vi "PS采集测试.vi"() -> ()   [LabVIEW 2020]
uses:
  <vilib>/DAQmx/read.llb/DAQmx Read (Counter 1D DBL 1Chan NSamp).vi
  <vilib>/DAQmx/read.llb/DAQmx Read (Counter DBL 1Chan 1Samp).vi
  <vilib>/DAQmx/create/channels.llb/DAQmx Create Channel (CI-Period).vi
  <vilib>/DAQmx/configure/timing.llb/DAQmx Timing (Implicit).vi
  <vilib>/DAQmx/miscellaneous.llb/DAQmx Fill In Error Info.vi
  <userlib>/_MGI/1D Array/MGI Average/MGI Average (DBL[]).vi
  <vilib>/DAQmx/create/channels.llb/DAQmx Create Channel (CI-Pulse Width).vi
  <resource>/objmgr/daqmx.rc
panel:
  out "周期 8":dbl
  out "周期 7":dbl
  out "周期 6":dbl
  out "周期 5":dbl
  out "周期 4":dbl
  out "周期 3":dbl
  out "占空比 8":dbl
  in  "通道 8":tag="Dev2/ctr7"
  out "占空比 7":dbl
  in  "通道 7":tag="Dev2/ctr6"
  out "占空比 6":dbl
  in  "通道 6":tag="Dev2/ctr5"
  out "占空比 5":dbl
  in  "通道 5":tag="Dev2/ctr4"
  out "占空比 4":dbl
  in  "通道 4":tag="Dev2/ctr3"
  out "占空比 3":dbl
  in  "通道 3":tag="Dev2/ctr2"
  out "周期 2":dbl
  out "占空比 2":dbl
  in  "通道 2":tag="Dev2/ctr1"
  in  "通道":tag="Dev2/ctr0"
  in  "停止":bool
  out "占空比":dbl
  out "周期":dbl
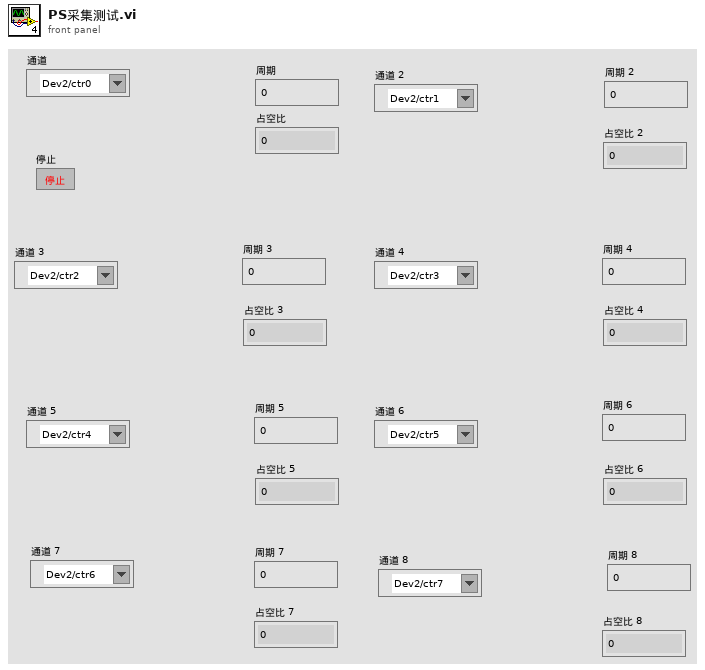
[diagram p1: front panel]
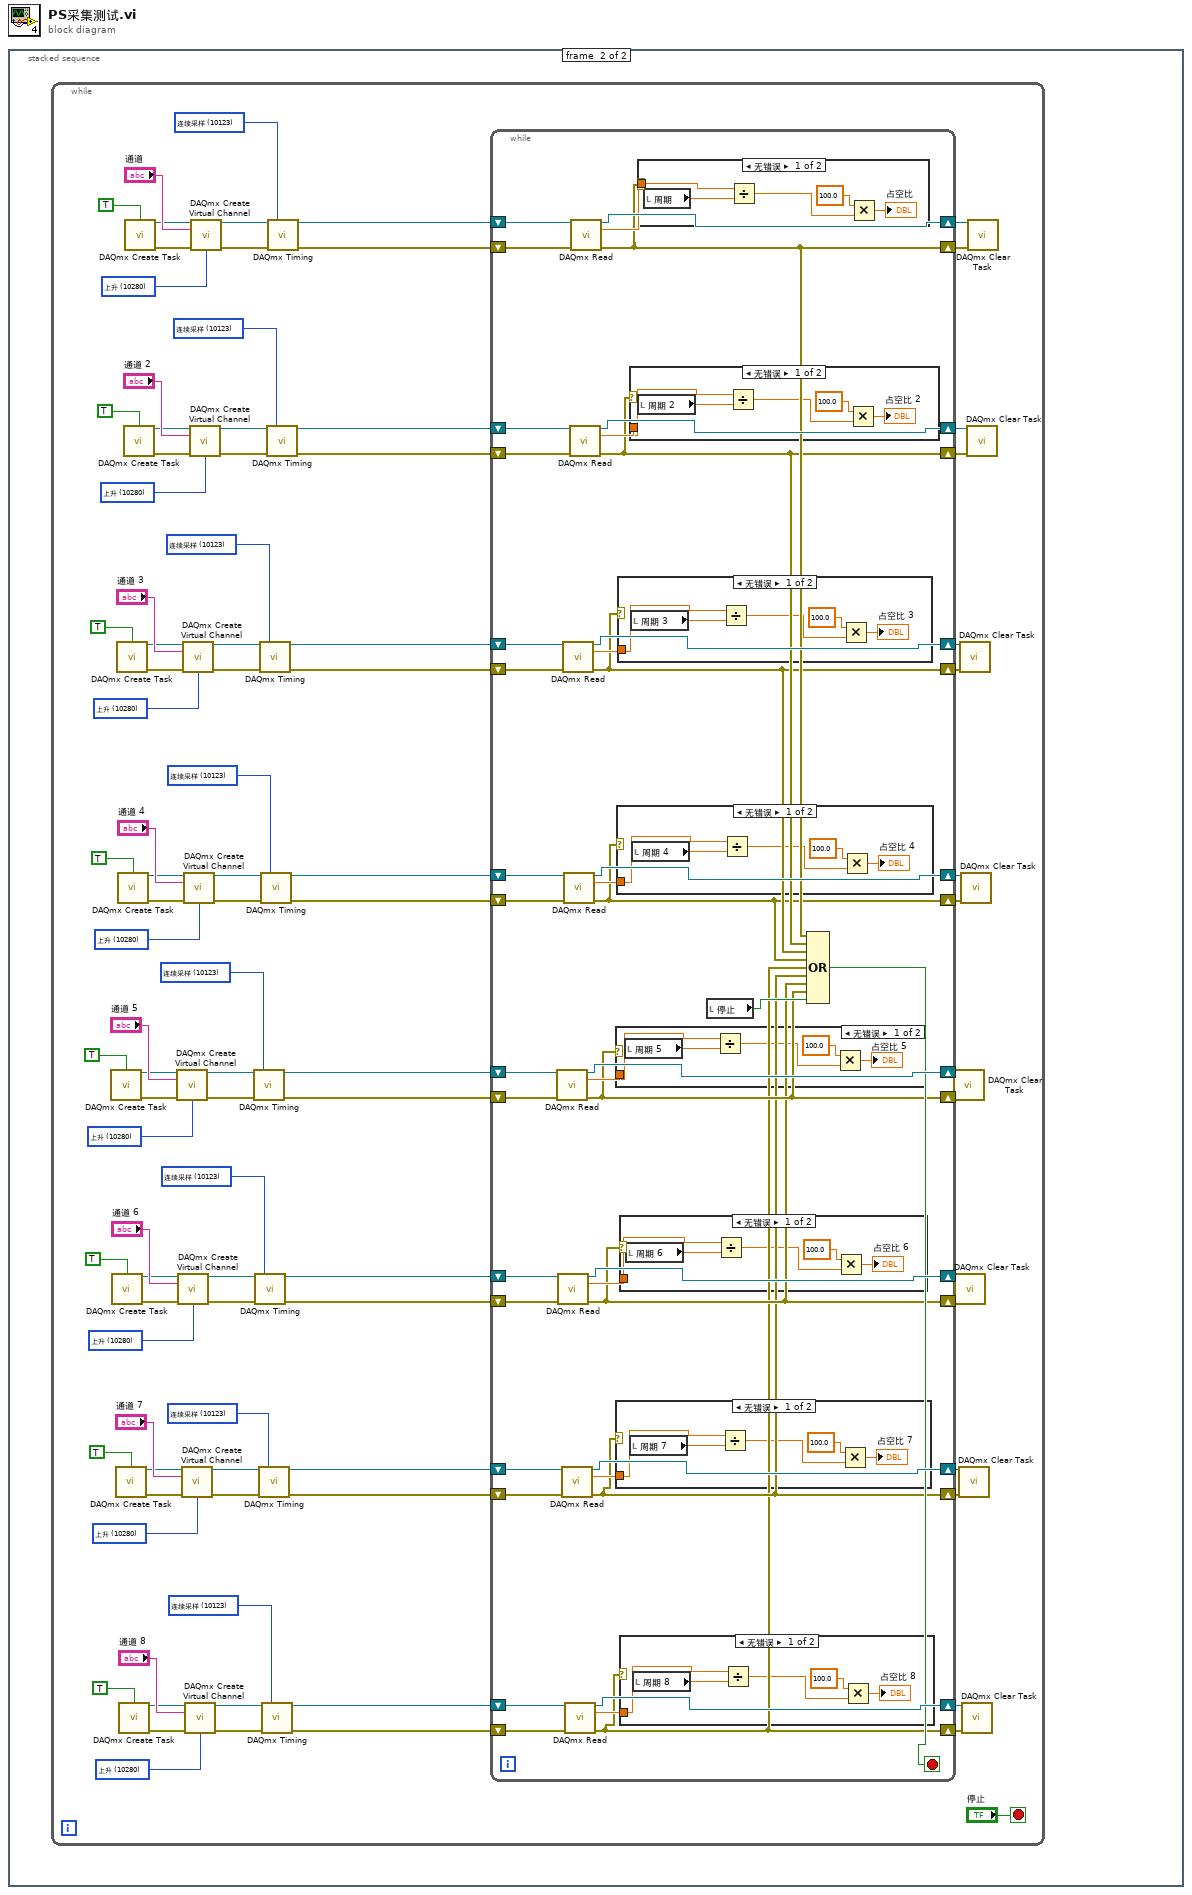
[diagram p0: block diagram]
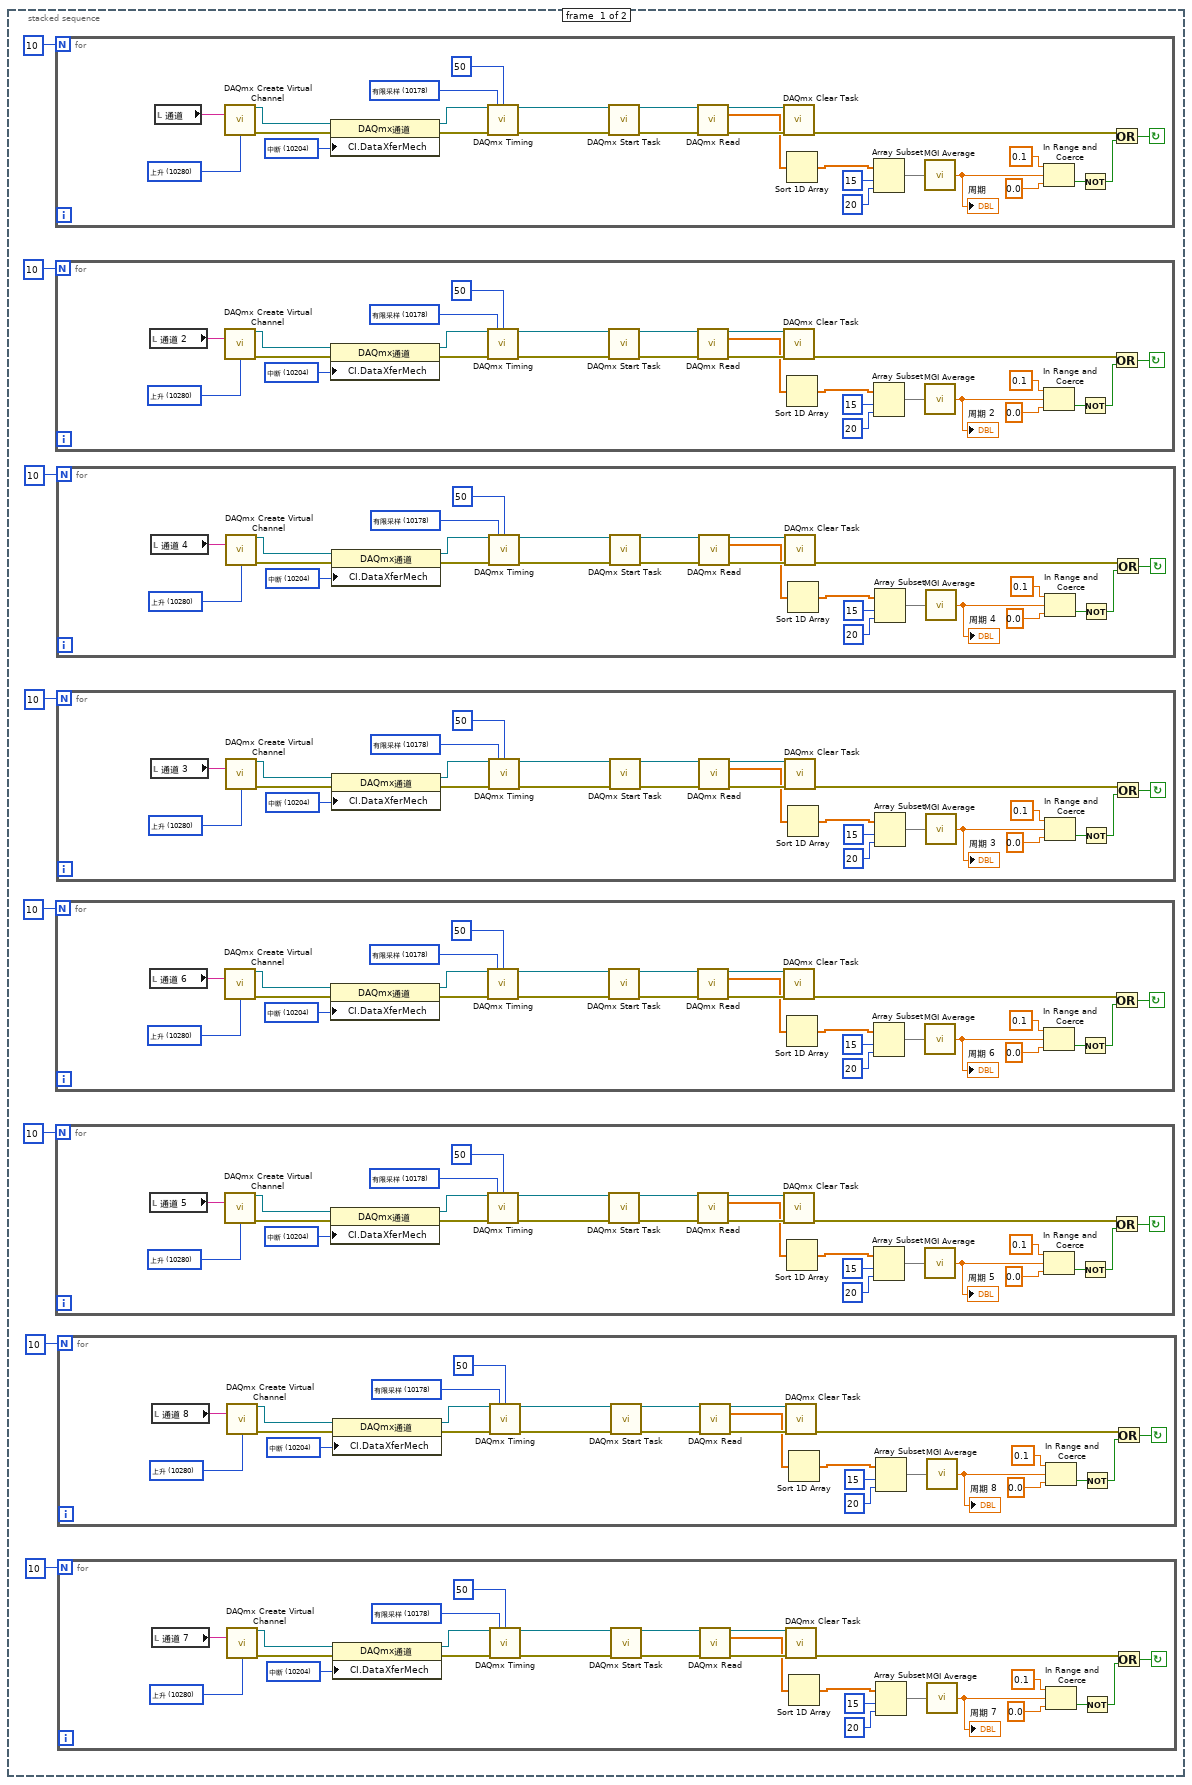
[diagram p2: hidden frame]
diagram:
  n1 = stacked-sequence {
    frame #0 {
      n2 = for {
        N: 10 -> [_]
        stop <- w200 continue-if-true
        w211 = 10204 items=["DMA"=10054, "中断"=10204, "程序控制I/O"=10264, "USB Bulk"=12590] ("CI.DataXferMech")
        w215 = 10178 items=["有限采样"=10178, "连续采样"=10123, "硬件定时单点"=12522] ("sample mode")
        w224 = 10280 items=["上升"=10280, "下降"=10171] ("starting edge")
        n3 = local read "通道"() -> (w198:tag)
        n4 = call-poly <vilib>:"DAQmx Create Virtual Channel.vi"("counter"=w198, "starting edge"=w224) -> ("task out"=w223:refnum<k21>, "error out"=w213:errorcluster)  [unwired: 12 in]
        n5 = property class="DAQmx通道"(reference=w223, error in=w213, "CI.DataXferMech"=w211) -> (reference out=w214:refnum<k21>, error out=w212:errorcluster)
        n6 = call-poly <vilib>:"DAQmx Timing.vi"("task/channels in"=w214, "sample mode"=w215, "samples per channel"=50, "error in"=w212) -> ("task out"=w222:refnum<k21>, "error out"=w221:errorcluster)  [unwired: 10 in]
        n7 = call <vilib>:"DAQmx Start Task.vi"("task/channels in"=w222, "error in"=w221) -> ("task out"=w220:refnum<k21>, "error out"=w219:errorcluster)  [unwired: 12 in]
        n8 = call-poly <vilib>:"DAQmx Read.vi"("task/channels in"=w220, "error in"=w219) -> ("task out"=w217:refnum<k21>, "data"=w207:dbl[], "error out"=w218:errorcluster)  [unwired: 11 in]
        n9 = call <vilib>:"DAQmx Clear Task.vi"("task in"=w217, "error in"=w218) -> ("error out"=w203:errorcluster)  [unwired: 13 in]
        n10 = Sort 1D Array(array=w207) -> (sorted array=w210:dbl[])
        n11 = Array Subset(array=w210, index=15 ("索引"), length=20 ("长度")) -> (w199:dbl[])
        n12 = call-poly <userlib>:"MGI Average.vi"("Double[]"=w199) -> ("Average"=w204:dbl)  [unwired: 1 in]
        "周期" <- w204
        n13 = In Range and Coerce(upper limit=0.1 ("上限"), x=w204, lower limit=0.0 ("上限")) -> (In Range?=w202:bool)  [unwired: 1 out]
        n14 = Not(x=w202) -> (.not. x?=w201:bool)
        n15 = Or(x=w203, y=w201) -> (x .or. y?=w200:bool)
      }
      n16 = for {
        N: 10 -> [_]
        stop <- w173 continue-if-true
        w184 = 10204 items=["DMA"=10054, "中断"=10204, "程序控制I/O"=10264, "USB Bulk"=12590] ("CI.DataXferMech")
        w188 = 10178 items=["有限采样"=10178, "连续采样"=10123, "硬件定时单点"=12522] ("sample mode")
        w197 = 10280 items=["上升"=10280, "下降"=10171] ("starting edge")
        n17 = local read "通道 2"() -> (w171:tag)
        n18 = call-poly <vilib>:"DAQmx Create Virtual Channel.vi"("counter"=w171, "starting edge"=w197) -> ("task out"=w196:refnum<k21>, "error out"=w186:errorcluster)  [unwired: 12 in]
        n19 = property class="DAQmx通道"(reference=w196, error in=w186, "CI.DataXferMech"=w184) -> (reference out=w187:refnum<k21>, error out=w185:errorcluster)
        n20 = call-poly <vilib>:"DAQmx Timing.vi"("task/channels in"=w187, "sample mode"=w188, "samples per channel"=50, "error in"=w185) -> ("task out"=w195:refnum<k21>, "error out"=w194:errorcluster)  [unwired: 10 in]
        n21 = call <vilib>:"DAQmx Start Task.vi"("task/channels in"=w195, "error in"=w194) -> ("task out"=w193:refnum<k21>, "error out"=w192:errorcluster)  [unwired: 12 in]
        n22 = call-poly <vilib>:"DAQmx Read.vi"("task/channels in"=w193, "error in"=w192) -> ("task out"=w190:refnum<k21>, "data"=w180:dbl[], "error out"=w191:errorcluster)  [unwired: 11 in]
        n23 = call <vilib>:"DAQmx Clear Task.vi"("task in"=w190, "error in"=w191) -> ("error out"=w176:errorcluster)  [unwired: 13 in]
        n24 = Sort 1D Array(array=w180) -> (sorted array=w183:dbl[])
        n25 = Array Subset(array=w183, index=15 ("索引"), length=20 ("长度")) -> (w172:dbl[])
        n26 = call-poly <userlib>:"MGI Average.vi"("Double[]"=w172) -> ("Average"=w177:dbl)  [unwired: 1 in]
        "周期 2" <- w177
        n27 = In Range and Coerce(upper limit=0.1 ("上限"), x=w177, lower limit=0.0 ("上限")) -> (In Range?=w175:bool)  [unwired: 1 out]
        n28 = Not(x=w175) -> (.not. x?=w174:bool)
        n29 = Or(x=w176, y=w174) -> (x .or. y?=w173:bool)
      }
      n30 = for {
        N: 10 -> [_]
        stop <- w92 continue-if-true
        w103 = 10204 items=["DMA"=10054, "中断"=10204, "程序控制I/O"=10264, "USB Bulk"=12590] ("CI.DataXferMech")
        w107 = 10178 items=["有限采样"=10178, "连续采样"=10123, "硬件定时单点"=12522] ("sample mode")
        w116 = 10280 items=["上升"=10280, "下降"=10171] ("starting edge")
        n31 = local read "通道 6"() -> (w90:tag)
        n32 = call-poly <vilib>:"DAQmx Create Virtual Channel.vi"("counter"=w90, "starting edge"=w116) -> ("task out"=w115:refnum<k21>, "error out"=w105:errorcluster)  [unwired: 12 in]
        n33 = property class="DAQmx通道"(reference=w115, error in=w105, "CI.DataXferMech"=w103) -> (reference out=w106:refnum<k21>, error out=w104:errorcluster)
        n34 = call-poly <vilib>:"DAQmx Timing.vi"("task/channels in"=w106, "sample mode"=w107, "samples per channel"=50, "error in"=w104) -> ("task out"=w114:refnum<k21>, "error out"=w113:errorcluster)  [unwired: 10 in]
        n35 = call <vilib>:"DAQmx Start Task.vi"("task/channels in"=w114, "error in"=w113) -> ("task out"=w112:refnum<k21>, "error out"=w111:errorcluster)  [unwired: 12 in]
        n36 = call-poly <vilib>:"DAQmx Read.vi"("task/channels in"=w112, "error in"=w111) -> ("task out"=w109:refnum<k21>, "data"=w99:dbl[], "error out"=w110:errorcluster)  [unwired: 11 in]
        n37 = call <vilib>:"DAQmx Clear Task.vi"("task in"=w109, "error in"=w110) -> ("error out"=w95:errorcluster)  [unwired: 13 in]
        n38 = Sort 1D Array(array=w99) -> (sorted array=w102:dbl[])
        n39 = Array Subset(array=w102, index=15 ("索引"), length=20 ("长度")) -> (w91:dbl[])
        n40 = call-poly <userlib>:"MGI Average.vi"("Double[]"=w91) -> ("Average"=w96:dbl)  [unwired: 1 in]
        "周期 6" <- w96
        n41 = In Range and Coerce(upper limit=0.1 ("上限"), x=w96, lower limit=0.0 ("上限")) -> (In Range?=w94:bool)  [unwired: 1 out]
        n42 = Not(x=w94) -> (.not. x?=w93:bool)
        n43 = Or(x=w95, y=w93) -> (x .or. y?=w92:bool)
      }
      n44 = for {
        N: 10 -> [_]
        stop <- w65 continue-if-true
        w76 = 10204 items=["DMA"=10054, "中断"=10204, "程序控制I/O"=10264, "USB Bulk"=12590] ("CI.DataXferMech")
        w80 = 10178 items=["有限采样"=10178, "连续采样"=10123, "硬件定时单点"=12522] ("sample mode")
        w89 = 10280 items=["上升"=10280, "下降"=10171] ("starting edge")
        n45 = local read "通道 5"() -> (w63:tag)
        n46 = call-poly <vilib>:"DAQmx Create Virtual Channel.vi"("counter"=w63, "starting edge"=w89) -> ("task out"=w88:refnum<k21>, "error out"=w78:errorcluster)  [unwired: 12 in]
        n47 = property class="DAQmx通道"(reference=w88, error in=w78, "CI.DataXferMech"=w76) -> (reference out=w79:refnum<k21>, error out=w77:errorcluster)
        n48 = call-poly <vilib>:"DAQmx Timing.vi"("task/channels in"=w79, "sample mode"=w80, "samples per channel"=50, "error in"=w77) -> ("task out"=w87:refnum<k21>, "error out"=w86:errorcluster)  [unwired: 10 in]
        n49 = call <vilib>:"DAQmx Start Task.vi"("task/channels in"=w87, "error in"=w86) -> ("task out"=w85:refnum<k21>, "error out"=w84:errorcluster)  [unwired: 12 in]
        n50 = call-poly <vilib>:"DAQmx Read.vi"("task/channels in"=w85, "error in"=w84) -> ("task out"=w82:refnum<k21>, "data"=w72:dbl[], "error out"=w83:errorcluster)  [unwired: 11 in]
        n51 = call <vilib>:"DAQmx Clear Task.vi"("task in"=w82, "error in"=w83) -> ("error out"=w68:errorcluster)  [unwired: 13 in]
        n52 = Sort 1D Array(array=w72) -> (sorted array=w75:dbl[])
        n53 = Array Subset(array=w75, index=15 ("索引"), length=20 ("长度")) -> (w64:dbl[])
        n54 = call-poly <userlib>:"MGI Average.vi"("Double[]"=w64) -> ("Average"=w69:dbl)  [unwired: 1 in]
        "周期 5" <- w69
        n55 = In Range and Coerce(upper limit=0.1 ("上限"), x=w69, lower limit=0.0 ("上限")) -> (In Range?=w67:bool)  [unwired: 1 out]
        n56 = Not(x=w67) -> (.not. x?=w66:bool)
        n57 = Or(x=w68, y=w66) -> (x .or. y?=w65:bool)
      }
      n58 = for {
        N: 10 -> [_]
        stop <- w146 continue-if-true
        w157 = 10204 items=["DMA"=10054, "中断"=10204, "程序控制I/O"=10264, "USB Bulk"=12590] ("CI.DataXferMech")
        w161 = 10178 items=["有限采样"=10178, "连续采样"=10123, "硬件定时单点"=12522] ("sample mode")
        w170 = 10280 items=["上升"=10280, "下降"=10171] ("starting edge")
        n59 = local read "通道 4"() -> (w144:tag)
        n60 = call-poly <vilib>:"DAQmx Create Virtual Channel.vi"("counter"=w144, "starting edge"=w170) -> ("task out"=w169:refnum<k21>, "error out"=w159:errorcluster)  [unwired: 12 in]
        n61 = property class="DAQmx通道"(reference=w169, error in=w159, "CI.DataXferMech"=w157) -> (reference out=w160:refnum<k21>, error out=w158:errorcluster)
        n62 = call-poly <vilib>:"DAQmx Timing.vi"("task/channels in"=w160, "sample mode"=w161, "samples per channel"=50, "error in"=w158) -> ("task out"=w168:refnum<k21>, "error out"=w167:errorcluster)  [unwired: 10 in]
        n63 = call <vilib>:"DAQmx Start Task.vi"("task/channels in"=w168, "error in"=w167) -> ("task out"=w166:refnum<k21>, "error out"=w165:errorcluster)  [unwired: 12 in]
        n64 = call-poly <vilib>:"DAQmx Read.vi"("task/channels in"=w166, "error in"=w165) -> ("task out"=w163:refnum<k21>, "data"=w153:dbl[], "error out"=w164:errorcluster)  [unwired: 11 in]
        n65 = call <vilib>:"DAQmx Clear Task.vi"("task in"=w163, "error in"=w164) -> ("error out"=w149:errorcluster)  [unwired: 13 in]
        n66 = Sort 1D Array(array=w153) -> (sorted array=w156:dbl[])
        n67 = Array Subset(array=w156, index=15 ("索引"), length=20 ("长度")) -> (w145:dbl[])
        n68 = call-poly <userlib>:"MGI Average.vi"("Double[]"=w145) -> ("Average"=w150:dbl)  [unwired: 1 in]
        "周期 4" <- w150
        n69 = In Range and Coerce(upper limit=0.1 ("上限"), x=w150, lower limit=0.0 ("上限")) -> (In Range?=w148:bool)  [unwired: 1 out]
        n70 = Not(x=w148) -> (.not. x?=w147:bool)
        n71 = Or(x=w149, y=w147) -> (x .or. y?=w146:bool)
      }
      n72 = for {
        N: 10 -> [_]
        stop <- w119 continue-if-true
        w130 = 10204 items=["DMA"=10054, "中断"=10204, "程序控制I/O"=10264, "USB Bulk"=12590] ("CI.DataXferMech")
        w134 = 10178 items=["有限采样"=10178, "连续采样"=10123, "硬件定时单点"=12522] ("sample mode")
        w143 = 10280 items=["上升"=10280, "下降"=10171] ("starting edge")
        n73 = local read "通道 3"() -> (w117:tag)
        n74 = call-poly <vilib>:"DAQmx Create Virtual Channel.vi"("counter"=w117, "starting edge"=w143) -> ("task out"=w142:refnum<k21>, "error out"=w132:errorcluster)  [unwired: 12 in]
        n75 = property class="DAQmx通道"(reference=w142, error in=w132, "CI.DataXferMech"=w130) -> (reference out=w133:refnum<k21>, error out=w131:errorcluster)
        n76 = call-poly <vilib>:"DAQmx Timing.vi"("task/channels in"=w133, "sample mode"=w134, "samples per channel"=50, "error in"=w131) -> ("task out"=w141:refnum<k21>, "error out"=w140:errorcluster)  [unwired: 10 in]
        n77 = call <vilib>:"DAQmx Start Task.vi"("task/channels in"=w141, "error in"=w140) -> ("task out"=w139:refnum<k21>, "error out"=w138:errorcluster)  [unwired: 12 in]
        n78 = call-poly <vilib>:"DAQmx Read.vi"("task/channels in"=w139, "error in"=w138) -> ("task out"=w136:refnum<k21>, "data"=w126:dbl[], "error out"=w137:errorcluster)  [unwired: 11 in]
        n79 = call <vilib>:"DAQmx Clear Task.vi"("task in"=w136, "error in"=w137) -> ("error out"=w122:errorcluster)  [unwired: 13 in]
        n80 = Sort 1D Array(array=w126) -> (sorted array=w129:dbl[])
        n81 = Array Subset(array=w129, index=15 ("索引"), length=20 ("长度")) -> (w118:dbl[])
        n82 = call-poly <userlib>:"MGI Average.vi"("Double[]"=w118) -> ("Average"=w123:dbl)  [unwired: 1 in]
        "周期 3" <- w123
        n83 = In Range and Coerce(upper limit=0.1 ("上限"), x=w123, lower limit=0.0 ("上限")) -> (In Range?=w121:bool)  [unwired: 1 out]
        n84 = Not(x=w121) -> (.not. x?=w120:bool)
        n85 = Or(x=w122, y=w120) -> (x .or. y?=w119:bool)
      }
      n86 = for {
        N: 10 -> [_]
        stop <- w38 continue-if-true
        w49 = 10204 items=["DMA"=10054, "中断"=10204, "程序控制I/O"=10264, "USB Bulk"=12590] ("CI.DataXferMech")
        w53 = 10178 items=["有限采样"=10178, "连续采样"=10123, "硬件定时单点"=12522] ("sample mode")
        w62 = 10280 items=["上升"=10280, "下降"=10171] ("starting edge")
        n87 = local read "通道 8"() -> (w36:tag)
        n88 = call-poly <vilib>:"DAQmx Create Virtual Channel.vi"("counter"=w36, "starting edge"=w62) -> ("task out"=w61:refnum<k21>, "error out"=w51:errorcluster)  [unwired: 12 in]
        n89 = property class="DAQmx通道"(reference=w61, error in=w51, "CI.DataXferMech"=w49) -> (reference out=w52:refnum<k21>, error out=w50:errorcluster)
        n90 = call-poly <vilib>:"DAQmx Timing.vi"("task/channels in"=w52, "sample mode"=w53, "samples per channel"=50, "error in"=w50) -> ("task out"=w60:refnum<k21>, "error out"=w59:errorcluster)  [unwired: 10 in]
        n91 = call <vilib>:"DAQmx Start Task.vi"("task/channels in"=w60, "error in"=w59) -> ("task out"=w58:refnum<k21>, "error out"=w57:errorcluster)  [unwired: 12 in]
        n92 = call-poly <vilib>:"DAQmx Read.vi"("task/channels in"=w58, "error in"=w57) -> ("task out"=w55:refnum<k21>, "data"=w45:dbl[], "error out"=w56:errorcluster)  [unwired: 11 in]
        n93 = call <vilib>:"DAQmx Clear Task.vi"("task in"=w55, "error in"=w56) -> ("error out"=w41:errorcluster)  [unwired: 13 in]
        n94 = Sort 1D Array(array=w45) -> (sorted array=w48:dbl[])
        n95 = Array Subset(array=w48, index=15 ("索引"), length=20 ("长度")) -> (w37:dbl[])
        n96 = call-poly <userlib>:"MGI Average.vi"("Double[]"=w37) -> ("Average"=w42:dbl)  [unwired: 1 in]
        "周期 8" <- w42
        n97 = In Range and Coerce(upper limit=0.1 ("上限"), x=w42, lower limit=0.0 ("上限")) -> (In Range?=w40:bool)  [unwired: 1 out]
        n98 = Not(x=w40) -> (.not. x?=w39:bool)
        n99 = Or(x=w41, y=w39) -> (x .or. y?=w38:bool)
      }
      n100 = for {
        N: 10 -> [_]
        stop <- w11 continue-if-true
        w22 = 10204 items=["DMA"=10054, "中断"=10204, "程序控制I/O"=10264, "USB Bulk"=12590] ("CI.DataXferMech")
        w26 = 10178 items=["有限采样"=10178, "连续采样"=10123, "硬件定时单点"=12522] ("sample mode")
        w35 = 10280 items=["上升"=10280, "下降"=10171] ("starting edge")
        n101 = local read "通道 7"() -> (w9:tag)
        n102 = call-poly <vilib>:"DAQmx Create Virtual Channel.vi"("counter"=w9, "starting edge"=w35) -> ("task out"=w34:refnum<k21>, "error out"=w24:errorcluster)  [unwired: 12 in]
        n103 = property class="DAQmx通道"(reference=w34, error in=w24, "CI.DataXferMech"=w22) -> (reference out=w25:refnum<k21>, error out=w23:errorcluster)
        n104 = call-poly <vilib>:"DAQmx Timing.vi"("task/channels in"=w25, "sample mode"=w26, "samples per channel"=50, "error in"=w23) -> ("task out"=w33:refnum<k21>, "error out"=w32:errorcluster)  [unwired: 10 in]
        n105 = call <vilib>:"DAQmx Start Task.vi"("task/channels in"=w33, "error in"=w32) -> ("task out"=w31:refnum<k21>, "error out"=w30:errorcluster)  [unwired: 12 in]
        n106 = call-poly <vilib>:"DAQmx Read.vi"("task/channels in"=w31, "error in"=w30) -> ("task out"=w28:refnum<k21>, "data"=w18:dbl[], "error out"=w29:errorcluster)  [unwired: 11 in]
        n107 = call <vilib>:"DAQmx Clear Task.vi"("task in"=w28, "error in"=w29) -> ("error out"=w14:errorcluster)  [unwired: 13 in]
        n108 = Sort 1D Array(array=w18) -> (sorted array=w21:dbl[])
        n109 = Array Subset(array=w21, index=15 ("索引"), length=20 ("长度")) -> (w10:dbl[])
        n110 = call-poly <userlib>:"MGI Average.vi"("Double[]"=w10) -> ("Average"=w15:dbl)  [unwired: 1 in]
        "周期 7" <- w15
        n111 = In Range and Coerce(upper limit=0.1 ("上限"), x=w15, lower limit=0.0 ("上限")) -> (In Range?=w13:bool)  [unwired: 1 out]
        n112 = Not(x=w13) -> (.not. x?=w12:bool)
        n113 = Or(x=w14, y=w12) -> (x .or. y?=w11:bool)
      }
    }
    frame #1 {
      n114 = while {
        stop <- "停止" stop-if-true
        w231 = 10123 items=["有限采样"=10178, "连续采样"=10123, "硬件定时单点"=12522] ("sample mode")
        w230 = 10280 items=["上升"=10280, "下降"=10171] ("starting edge")
        w243 = 10123 items=["有限采样"=10178, "连续采样"=10123, "硬件定时单点"=12522] ("sample mode")
        w242 = 10280 items=["上升"=10280, "下降"=10171] ("starting edge")
        w255 = 10123 items=["有限采样"=10178, "连续采样"=10123, "硬件定时单点"=12522] ("sample mode")
        w254 = 10280 items=["上升"=10280, "下降"=10171] ("starting edge")
        w267 = 10123 items=["有限采样"=10178, "连续采样"=10123, "硬件定时单点"=12522] ("sample mode")
        w266 = 10280 items=["上升"=10280, "下降"=10171] ("starting edge")
        w279 = 10123 items=["有限采样"=10178, "连续采样"=10123, "硬件定时单点"=12522] ("sample mode")
        w278 = 10280 items=["上升"=10280, "下降"=10171] ("starting edge")
        w291 = 10123 items=["有限采样"=10178, "连续采样"=10123, "硬件定时单点"=12522] ("sample mode")
        w290 = 10280 items=["上升"=10280, "下降"=10171] ("starting edge")
        w303 = 10123 items=["有限采样"=10178, "连续采样"=10123, "硬件定时单点"=12522] ("sample mode")
        w302 = 10280 items=["上升"=10280, "下降"=10171] ("starting edge")
        w315 = 10123 items=["有限采样"=10178, "连续采样"=10123, "硬件定时单点"=12522] ("sample mode")
        w314 = 10280 items=["上升"=10280, "下降"=10171] ("starting edge")
        n115 = call <vilib>:"DAQmx Create Task.vi"("auto cleanup"=TRUE) -> ("task out"=w252:refnum<k21>, "error out"=w250:errorcluster)  [unwired: 13 in]
        n116 = call <vilib>:"DAQmx Create Task.vi"("auto cleanup"=TRUE) -> ("task out"=w264:refnum<k21>, "error out"=w262:errorcluster)  [unwired: 13 in]
        n117 = call <vilib>:"DAQmx Create Task.vi"("auto cleanup"=TRUE) -> ("task out"=w228:refnum<k21>, "error out"=w226:errorcluster)  [unwired: 13 in]
        n118 = call <vilib>:"DAQmx Create Task.vi"("auto cleanup"=TRUE) -> ("task out"=w288:refnum<k21>, "error out"=w286:errorcluster)  [unwired: 13 in]
        n119 = call <vilib>:"DAQmx Create Task.vi"("auto cleanup"=TRUE) -> ("task out"=w276:refnum<k21>, "error out"=w274:errorcluster)  [unwired: 13 in]
        n120 = call <vilib>:"DAQmx Create Task.vi"("auto cleanup"=TRUE) -> ("task out"=w240:refnum<k21>, "error out"=w238:errorcluster)  [unwired: 13 in]
        n121 = call <vilib>:"DAQmx Create Task.vi"("auto cleanup"=TRUE) -> ("task out"=w300:refnum<k21>, "error out"=w298:errorcluster)  [unwired: 13 in]
        n122 = call <vilib>:"DAQmx Create Task.vi"("auto cleanup"=TRUE) -> ("task out"=w312:refnum<k21>, "error out"=w310:errorcluster)  [unwired: 13 in]
        n123 = call-poly <vilib>:"DAQmx Create Virtual Channel.vi"("task in"=w252, "counter"="通道 5", "error in"=w250, "starting edge"=w254) -> ("task out"=w256:refnum<k21>, "error out"=w261:errorcluster)  [unwired: 10 in]
        n124 = call-poly <vilib>:"DAQmx Create Virtual Channel.vi"("task in"=w264, "counter"="通道 6", "error in"=w262, "starting edge"=w266) -> ("task out"=w268:refnum<k21>, "error out"=w273:errorcluster)  [unwired: 10 in]
        n125 = call-poly <vilib>:"DAQmx Create Virtual Channel.vi"("task in"=w228, "counter"="通道 7", "error in"=w226, "starting edge"=w230) -> ("task out"=w232:refnum<k21>, "error out"=w237:errorcluster)  [unwired: 10 in]
        n126 = call-poly <vilib>:"DAQmx Create Virtual Channel.vi"("task in"=w288, "counter"="通道 3", "error in"=w286, "starting edge"=w290) -> ("task out"=w292:refnum<k21>, "error out"=w297:errorcluster)  [unwired: 10 in]
        n127 = call-poly <vilib>:"DAQmx Create Virtual Channel.vi"("task in"=w276, "counter"="通道 4", "error in"=w274, "starting edge"=w278) -> ("task out"=w280:refnum<k21>, "error out"=w285:errorcluster)  [unwired: 10 in]
        n128 = call-poly <vilib>:"DAQmx Create Virtual Channel.vi"("task in"=w240, "counter"="通道 8", "error in"=w238, "starting edge"=w242) -> ("task out"=w244:refnum<k21>, "error out"=w249:errorcluster)  [unwired: 10 in]
        n129 = call-poly <vilib>:"DAQmx Create Virtual Channel.vi"("task in"=w300, "counter"="通道 2", "error in"=w298, "starting edge"=w302) -> ("task out"=w304:refnum<k21>, "error out"=w309:errorcluster)  [unwired: 10 in]
        n130 = call-poly <vilib>:"DAQmx Create Virtual Channel.vi"("task in"=w312, "counter"="通道", "error in"=w310, "starting edge"=w314) -> ("task out"=w316:refnum<k21>, "error out"=w321:errorcluster)  [unwired: 10 in]
        n131 = call-poly <vilib>:"DAQmx Timing.vi"("task/channels in"=w256, "sample mode"=w255, "error in"=w261) -> ("task out"=w257:refnum<k21>, "error out"=w258:errorcluster)  [unwired: 11 in]
        n132 = call-poly <vilib>:"DAQmx Timing.vi"("task/channels in"=w268, "sample mode"=w267, "error in"=w273) -> ("task out"=w269:refnum<k21>, "error out"=w270:errorcluster)  [unwired: 11 in]
        n133 = call-poly <vilib>:"DAQmx Timing.vi"("task/channels in"=w232, "sample mode"=w231, "error in"=w237) -> ("task out"=w233:refnum<k21>, "error out"=w234:errorcluster)  [unwired: 11 in]
        n134 = call-poly <vilib>:"DAQmx Timing.vi"("task/channels in"=w292, "sample mode"=w291, "error in"=w297) -> ("task out"=w293:refnum<k21>, "error out"=w294:errorcluster)  [unwired: 11 in]
        n135 = call-poly <vilib>:"DAQmx Timing.vi"("task/channels in"=w280, "sample mode"=w279, "error in"=w285) -> ("task out"=w281:refnum<k21>, "error out"=w282:errorcluster)  [unwired: 11 in]
        n136 = call-poly <vilib>:"DAQmx Timing.vi"("task/channels in"=w244, "sample mode"=w243, "error in"=w249) -> ("task out"=w245:refnum<k21>, "error out"=w246:errorcluster)  [unwired: 11 in]
        n137 = call-poly <vilib>:"DAQmx Timing.vi"("task/channels in"=w304, "sample mode"=w303, "error in"=w309) -> ("task out"=w305:refnum<k21>, "error out"=w306:errorcluster)  [unwired: 11 in]
        n138 = call-poly <vilib>:"DAQmx Timing.vi"("task/channels in"=w316, "sample mode"=w315, "error in"=w321) -> ("task out"=w317:refnum<k21>, "error out"=w318:errorcluster)  [unwired: 11 in]
        n139 = while {
          shift-right: [w329] -> w319
          shift-left: w318 -> [w362]
          shift-right: [w363] -> w320
          shift-left: w317 -> [w361]
          shift-right: [w328] -> w307
          shift-left: w306 -> [w359]
          shift-right: [w360] -> w308
          shift-left: w305 -> [w358]
          shift-right: [w327] -> w295
          shift-left: w294 -> [w356]
          shift-right: [w357] -> w296
          shift-left: w293 -> [w355]
          shift-right: [w326] -> w283
          shift-left: w282 -> [w353]
          shift-right: [w354] -> w284
          shift-left: w281 -> [w352]
          shift-right: [w324] -> w271
          shift-left: w270 -> [w350]
          shift-right: [w351] -> w272
          shift-left: w269 -> [w349]
          shift-right: [w325] -> w259
          shift-left: w258 -> [w347]
          shift-right: [w348] -> w260
          shift-left: w257 -> [w346]
          shift-right: [w322] -> w247
          shift-left: w246 -> [w344]
          shift-right: [w345] -> w248
          shift-left: w245 -> [w343]
          shift-right: [w323] -> w235
          shift-left: w234 -> [w341]
          shift-right: [w342] -> w236
          shift-left: w233 -> [w340]
          stop <- w330 stop-if-true
          n140 = call-poly <vilib>:"DAQmx Read.vi"("task/channels in"=w346, "error in"=w347) -> ("task out"=w348:refnum<k21>, "data"=w334:dbl, "error out"=w325:errorcluster)  [unwired: 11 in]
          n141 = call-poly <vilib>:"DAQmx Read.vi"("task/channels in"=w349, "error in"=w350) -> ("task out"=w351:refnum<k21>, "data"=w335:dbl, "error out"=w324:errorcluster)  [unwired: 11 in]
          n142 = call-poly <vilib>:"DAQmx Read.vi"("task/channels in"=w340, "error in"=w341) -> ("task out"=w342:refnum<k21>, "data"=w332:dbl, "error out"=w323:errorcluster)  [unwired: 11 in]
          n143 = call-poly <vilib>:"DAQmx Read.vi"("task/channels in"=w355, "error in"=w356) -> ("task out"=w357:refnum<k21>, "data"=w337:dbl, "error out"=w327:errorcluster)  [unwired: 11 in]
          n144 = call-poly <vilib>:"DAQmx Read.vi"("task/channels in"=w352, "error in"=w353) -> ("task out"=w354:refnum<k21>, "data"=w336:dbl, "error out"=w326:errorcluster)  [unwired: 11 in]
          n145 = call-poly <vilib>:"DAQmx Read.vi"("task/channels in"=w343, "error in"=w344) -> ("task out"=w345:refnum<k21>, "data"=w333:dbl, "error out"=w322:errorcluster)  [unwired: 11 in]
          n146 = call-poly <vilib>:"DAQmx Read.vi"("task/channels in"=w358, "error in"=w359) -> ("task out"=w360:refnum<k21>, "data"=w338:dbl, "error out"=w328:errorcluster)  [unwired: 11 in]
          n147 = call-poly <vilib>:"DAQmx Read.vi"("task/channels in"=w361, "error in"=w362) -> ("task out"=w363:refnum<k21>, "data"=w339:dbl, "error out"=w329:errorcluster)  [unwired: 11 in]
          n148 = case shown="无错误" w325 {
            tunnel: w334 -> [w383 _]
            frame No Error {
              n149 = local read "周期 5"() -> (w382:dbl)
              n150 = Divide(x=w383, y=w382) -> (x/y=w381:dbl)
              n151 = Multiply(x=100.0, y=w381) -> (x*y=→"占空比 5":dbl)
            }
            frame Error {
            }
          }
          n152 = case shown="无错误" w323 {
            tunnel: w332 -> [w373 _]
            frame No Error {
              n153 = local read "周期 7"() -> (w372:dbl)
              n154 = Divide(x=w373, y=w372) -> (x/y=w371:dbl)
              n155 = Multiply(x=100.0, y=w371) -> (x*y=→"占空比 7":dbl)
            }
            frame Error {
            }
          }
          n156 = case shown="无错误" w326 {
            tunnel: w336 -> [w388 _]
            frame No Error {
              n157 = local read "周期 4"() -> (w387:dbl)
              n158 = Divide(x=w388, y=w387) -> (x/y=w386:dbl)
              n159 = Multiply(x=100.0, y=w386) -> (x*y=→"占空比 4":dbl)
            }
            frame Error {
            }
          }
          n160 = case shown="无错误" w327 {
            tunnel: w337 -> [w393 _]
            frame No Error {
              n161 = local read "周期 3"() -> (w392:dbl)
              n162 = Divide(x=w393, y=w392) -> (x/y=w391:dbl)
              n163 = Multiply(x=100.0, y=w391) -> (x*y=→"占空比 3":dbl)
            }
            frame Error {
            }
          }
          n164 = case shown="无错误" w324 {
            tunnel: w335 -> [w378 _]
            frame No Error {
              n165 = local read "周期 6"() -> (w377:dbl)
              n166 = Divide(x=w378, y=w377) -> (x/y=w376:dbl)
              n167 = Multiply(x=100.0, y=w376) -> (x*y=→"占空比 6":dbl)
            }
            frame Error {
            }
          }
          n168 = case shown="无错误" w322 {
            tunnel: w333 -> [w368 _]
            frame No Error {
              n169 = local read "周期 8"() -> (w367:dbl)
              n170 = Divide(x=w368, y=w367) -> (x/y=w366:dbl)
              n171 = Multiply(x=100.0, y=w366) -> (x*y=→"占空比 8":dbl)
            }
            frame Error {
            }
          }
          n172 = case shown="无错误" w328 {
            tunnel: w338 -> [w398 _]
            frame No Error {
              n173 = local read "周期 2"() -> (w397:dbl)
              n174 = Divide(x=w398, y=w397) -> (x/y=w396:dbl)
              n175 = Multiply(x=100.0, y=w396) -> (x*y=→"占空比 2":dbl)
            }
            frame Error {
            }
          }
          n176 = case shown="无错误" w329 {
            tunnel: w339 -> [w403 _]
            frame No Error {
              n177 = local read "周期"() -> (w402:dbl)
              n178 = Divide(x=w403, y=w402) -> (x/y=w401:dbl)
              n179 = Multiply(x=100.0, y=w401) -> (x*y=→"占空比":dbl)
            }
            frame Error {
            }
          }
          n180 = local read "停止"() -> (w331:bool)
          n181 = Compound Arithmetic op=OR ("复合运算")(w329, w328, w327, w326, w322, w323, w324, w325, w331) -> (w330:bool)
        }
        n182 = call <vilib>:"DAQmx Clear Task.vi"("task in"=w260, "error in"=w259) -> ()  [unwired: 13 in, 1 out]
        n183 = call <vilib>:"DAQmx Clear Task.vi"("task in"=w272, "error in"=w271) -> ()  [unwired: 13 in, 1 out]
        n184 = call <vilib>:"DAQmx Clear Task.vi"("task in"=w236, "error in"=w235) -> ()  [unwired: 13 in, 1 out]
        n185 = call <vilib>:"DAQmx Clear Task.vi"("task in"=w296, "error in"=w295) -> ()  [unwired: 13 in, 1 out]
        n186 = call <vilib>:"DAQmx Clear Task.vi"("task in"=w284, "error in"=w283) -> ()  [unwired: 13 in, 1 out]
        n187 = call <vilib>:"DAQmx Clear Task.vi"("task in"=w248, "error in"=w247) -> ()  [unwired: 13 in, 1 out]
        n188 = call <vilib>:"DAQmx Clear Task.vi"("task in"=w308, "error in"=w307) -> ()  [unwired: 13 in, 1 out]
        n189 = call <vilib>:"DAQmx Clear Task.vi"("task in"=w320, "error in"=w319) -> ()  [unwired: 13 in, 1 out]
      }
    }
  }
